vi "solar_voy_def Quotes Add LVType.vi"(9 "LVTYPE":T1, 10 "DESC in":string) -> (2 "DESC out":string)   [LabVIEW 2018]
doc: "This adds the custom LabVIEW data type to the COSMOS definition. Since COSMOS only supports UINT, INT, FLOAT, STRING and BLOCK. This allows Voyager to import the COSMOS definition file and determine the custom LabVIEW data types such as BOOLEAN, PATH, U8_ENUM..U64_ENUM, VISA and Arrays.\n\nEx: \"lv=BOOLEAN, My description is here\""
uses:
  type/solar_type Item Type.ctl
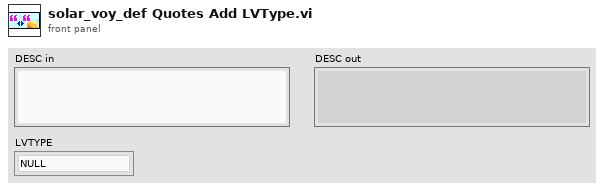
[diagram p1: front panel]
types:
  T1 = typedef "solar_type Item Type.ctl" = enum16{"NULL", "UNKNOWN", "CLUSTER", "I8", "I16", "I32", "I64", "U8", "U16", "U32", "U64", "U8_ENUM", "U16_ENUM", "U32_ENUM", "SGL", "DBL", "BOOLEAN", "STRING", "PATH", "VISA", "TAG", "TIME", "I8_1D", "I16_1D", "I32_1D", "I64_1D", "U8_1D", "U16_1D", "U32_1D", "U64_1D", "U8_ENUM_1D", "U16_ENUM_1D", "U32_ENUM_1D", "SGL_1D", "DBL_1D", "BOOLEAN_1D", "STRING_1D", "PATH_1D", "VISA_1D", "TAG_1D", "TIME_1D", "I8_2D", "I16_2D", "I32_2D", "I64_2D", "U8_2D", "U16_2D", "U32_2D", "U64_2D", "U8_ENUM_2D", "U16_ENUM_2D", "U32_ENUM_2D", "SGL_2D", "DBL_2D", "BOOLEAN_2D", "STRING_2D", "PATH_2D", "VISA_2D", "TAG_2D", "TIME_2D"}
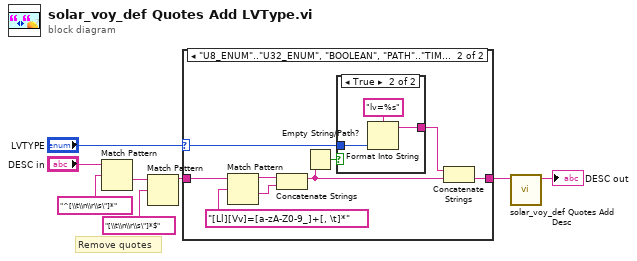
[diagram p0: block diagram]
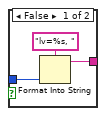
[diagram p3: hidden frame]
diagram:
  # "Remove quotes"
  n1 = Match Pattern(string="DESC in", regular expression="^[\\t\\n\\r\\s\"]*") -> (after substring=w3:string)  [unwired: 1 in, 3 out]
  n2 = Match Pattern(string=w3, regular expression="[\\t\\n\\r\\s\"]*$") -> (before substring=w7:string)  [unwired: 1 in, 3 out]
  n3 = case shown="\"U8_ENUM\"..\"U32_ENUM\", \"BOOLEAN\", \"PATH\"..\"TIME_2D\"" "LVTYPE" {
    selector: "LVTYPE" -> [_ w13]
    tunnel: w7 -> [w9 w18]
    tunnel: [w9 w10] -> w2
    frame "NULL".."U64", "SGL", "DBL", "STRING" {
    }
    frame "U8_ENUM".."U32_ENUM", "BOOLEAN", "PATH".."TIME_2D" {
      n4 = Match Pattern(string=w18, regular expression="[Ll][Vv]=[a-zA-Z0-9_]+[, \t]*") -> (before substring=w16:string, after substring=w15:string)  [unwired: 1 in, 2 out]
      n5 = Concatenate Strings(w16, w15) -> (w12:string)
      n6 = Empty String/Path?(string/path=w12) -> (empty?=w14:bool)
      n7 = case shown="True" w14 {
        tunnel: w13 -> [w20 w23]
        tunnel: [w19 w22] -> w11
        frame False {
          n8 = Format Into String(format string="lv=%s, ", w20) -> (resulting string=w19:string)  [unwired: 2 in, 1 out]
        }
        frame True {
          n9 = Format Into String(format string="lv=%s", w23) -> (resulting string=w22:string)  [unwired: 2 in, 1 out]
        }
      }
      n10 = Concatenate Strings(w11, w12) -> (w10:string)
    }
  }
  n11 = call "solar_voy_def Quotes Add Desc.vi"("Description"=w2) -> ("Description with Comments"=→"DESC out":string)  [unwired: 10 in]
